vi "DoubleClick.vi"(4 "Point":cluster{"H":T1, "V":T1}, 5 "XRef":refnum<vi>, 6 "State In":T2) -> (0 "Reply":string[](array[string]), 2 "State Out":T2)   [LabVIEW 2012]
doc: "This ability VI is called when the user double clicks on your XNode. Point is the the location on the XNode that the user clicked relative to the top-left corner of the XNode. A common pattern is to open a configuration dialog when the user double clicks on an XNode, but you may choose to behave differently. Use Reply to inform LabVIEW of any actions it needs to take.\n\nDefault behavior: None.\n\nThis ability provides UI and OS messages are handled."
uses:
  State.ctl
  <vilib>/XNodeSupport/XNodeInt.ctl
  FilterArray.xnode
  <vilib>/XNodeSupport/NI_XNodeSupport.lvlib
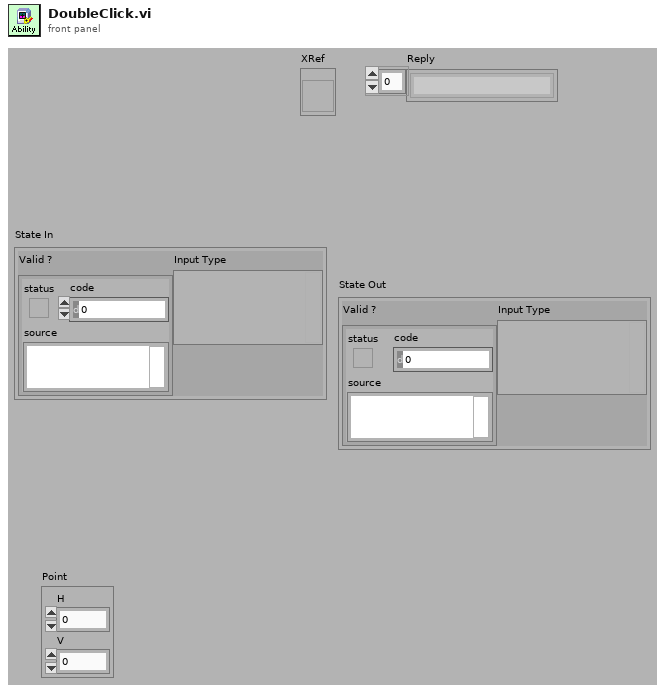
[diagram p1: front panel]
types:
  T1 = typedef "NI_XNodeSupport.lvlib/XNodeInt.ctl" = i32
  T2 = typedef "FilterArray.xnode/State.ctl" = cluster{"Valid ?":errorcluster, "Input Type":variant}
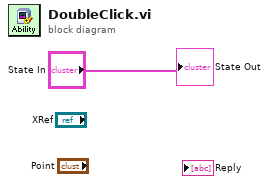
[diagram p0: block diagram]
diagram:
  "State Out" <- "State In"
